vi "MonitorZoomOffset.vi"() -> ()   [LabVIEW 2016]
uses:
  controls/Enum.ctl
  <vilib>/Utility/miscctls.llb/LVPointDoubleTypeDef.ctl
  Course Project/support/Message Queue/Message Cluster.ctl
  <vilib>/Utility/cursorutil.llb/Set Cursor (Icon Pict).vi
  Course Project/support/Message Queue/Message Queue.lvlib
panel:
  out "Line (um)":dbl format="%.2pm"
  in  "Square Zoom":bool
  in  "Apply Old":bool
  in  "Selection Old":T1(radio)
  out "Intensity Graph":dbl[][](graph)
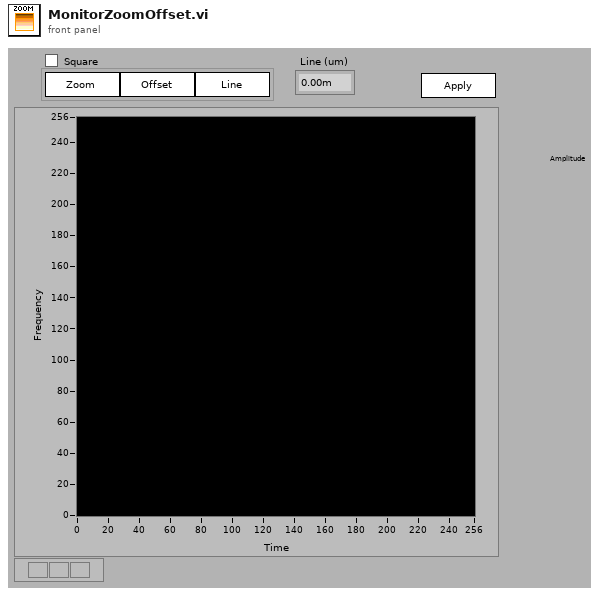
[diagram p1: front panel]
types:
  T1 = enum32{"No Selection", "Zoom", "Offset", "Profile\nProfile"}
  T2 = typedef "Enum.ctl" = enum16{"Init", "Read", "Write"}
  T3 = cluster{"Width":dbl, "Height":dbl, "X Offset":dbl, "Y Offset":dbl, "Angle":dbl, "Pixels/Line":u16, "Lines":u16, "Time/Line":dbl, "Scan Rate":dbl}
  T4 = typedef "LVRectTypeDef.ctl" = cluster{"Left":i16, "Top":i16, "Right":i16, "Bottom":i16}
  T5 = cluster{"Width":i16, "Style":enum32{"Solid", "Dash", "Dot", "DashDot", "DashDotDot"}}
  T6 = cluster{"Width":u16, "Style":enum32{"Solid", "Dash", "Dot", "DashDot", "DashDotDot"}}
  T7 = cluster{"left":i16, "top":i16, "right":i16, "bottom":i16}
  T8 = typedef "Message Queue.lvlib/Message Cluster.ctl" = cluster{"Message":string, "Données de message":variant}
  T9 = typedef "LVPoint32TypeDef.ctl" = cluster{"Horizontal":i32, "Vertical":i32}
  T10 = typedef "LVRangeTypeDef.ctl" = cluster{"Minimum":dbl, "Maximum":dbl, "Increment":dbl, "Minor Increment":dbl, "Start":dbl}
  T11 = typedef "LVBoundsTypeDef.ctl" = cluster{"Width":u32, "Height":u32}
  T12 = typedef "LVPointDoubleTypeDef.ctl" = cluster{"X":dbl, "Y":dbl}
  T13 = cluster{"Left coord px":dbl, "Right coord px":dbl, "Top coord px":dbl, "Bottom coord px":dbl}
  T14 = cluster{"Zoom Center  X um":dbl, "Zoom Center Y um":dbl}
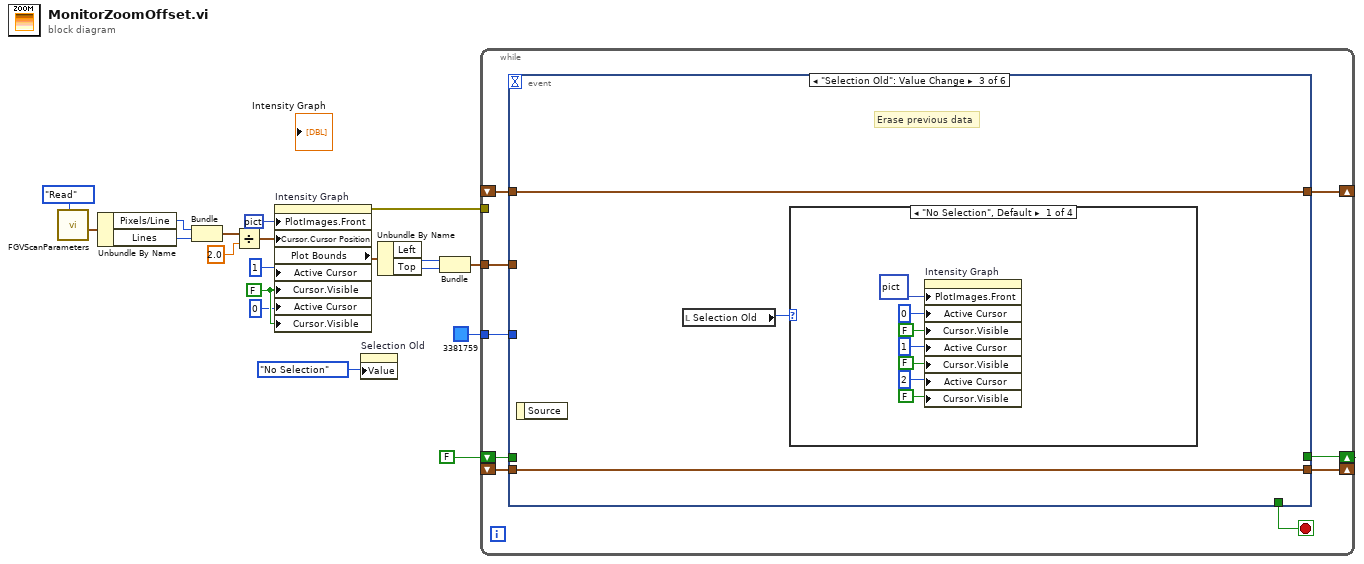
[diagram p0: block diagram]
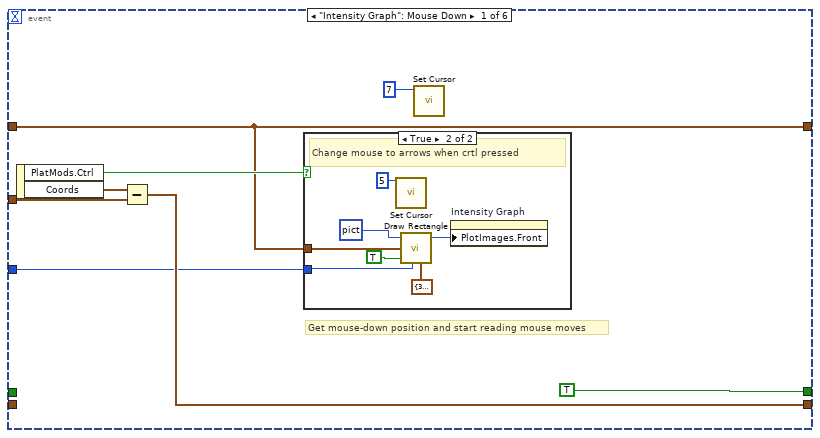
[diagram p2: hidden frame]
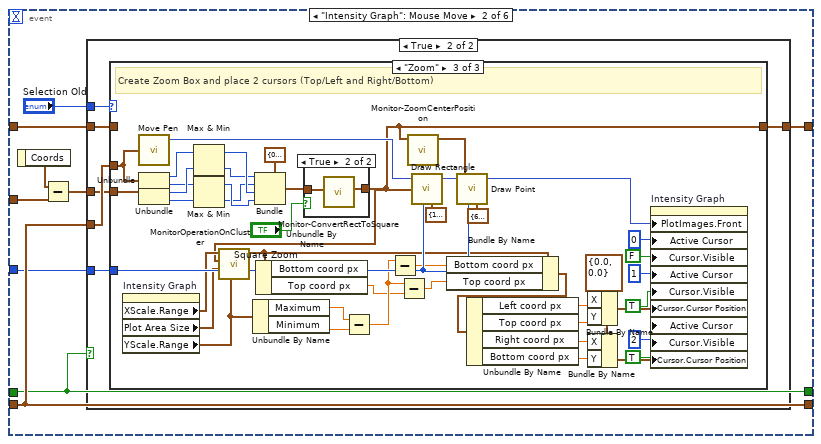
[diagram p4: hidden frame]
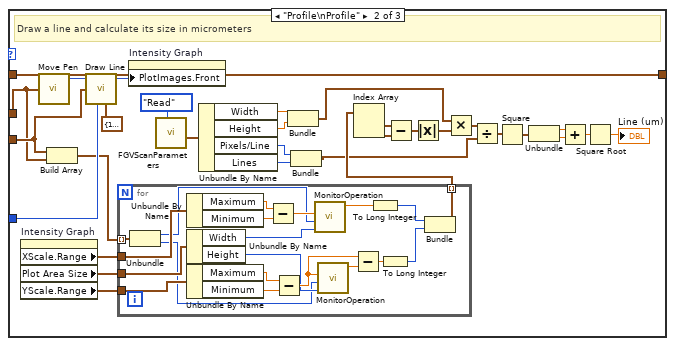
[diagram p7: hidden frame]
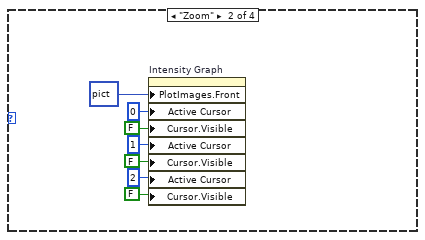
[diagram p9: hidden frame]
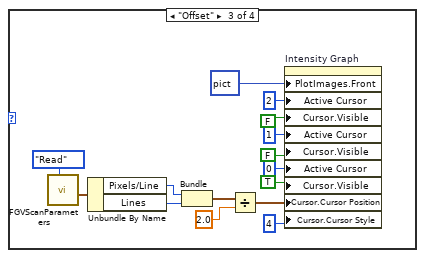
[diagram p10: hidden frame]
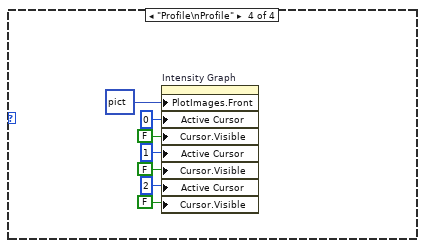
[diagram p11: hidden frame]
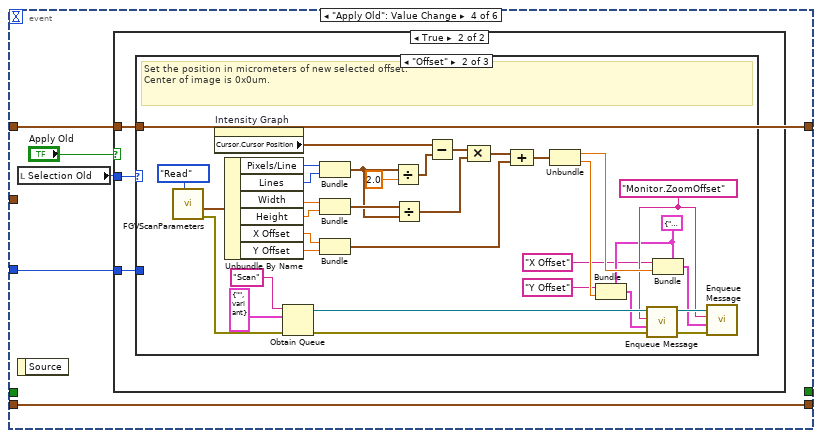
[diagram p12: hidden frame]
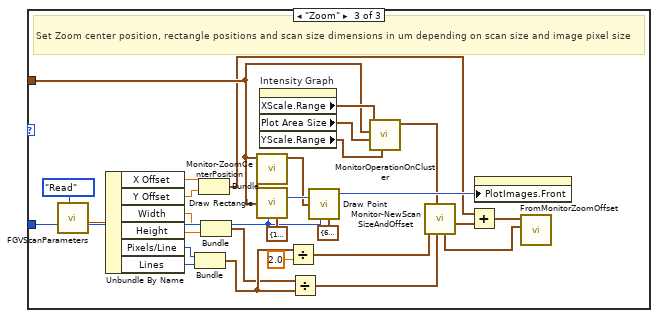
[diagram p15: hidden frame]
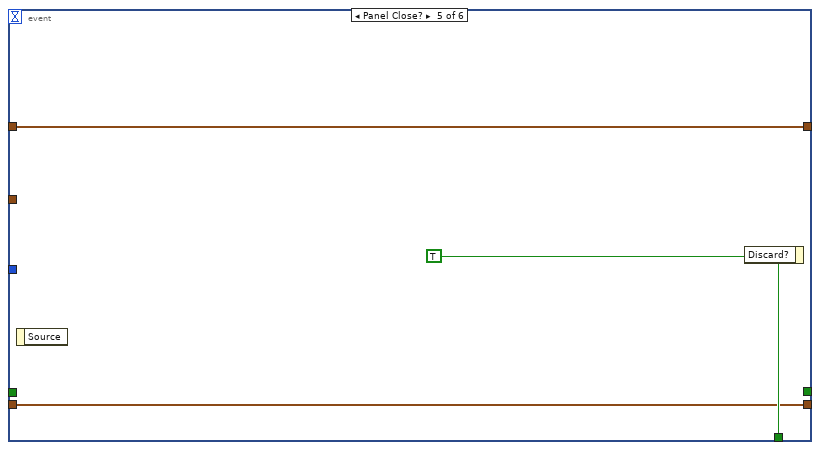
[diagram p16: hidden frame]
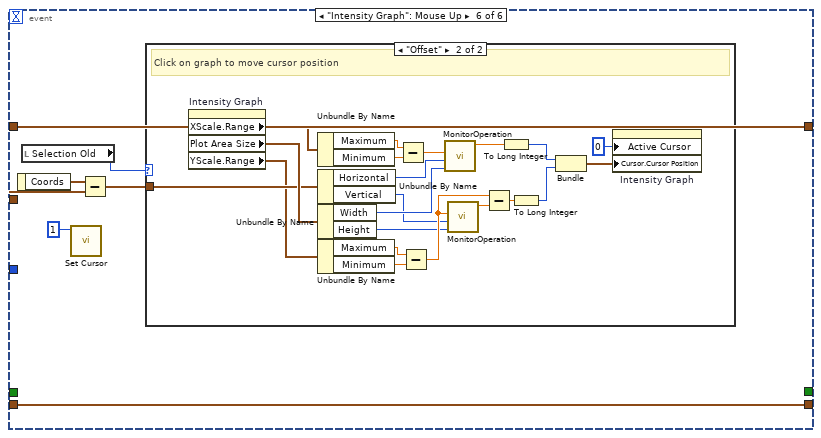
[diagram p17: hidden frame]
diagram:
  w7 = FALSE ("Cursor.Visible")
  n1 = call "FGVScanParameters.vi"("Enum"=Enum."Read") -> ("Scan Parameters Out"=w4:T3)  [unwired: 9 in, 1 out]
  n2 = Unbundle By Name(w4) -> ("Pixels/Line"=w3:u16, "Lines"=w2:u16)
  n3 = Bundle("Pixels/Line"=w3, "Lines"=w2) -> (w1:cluster{"Pixels/Line":u16, "Lines":u16})  [unwired: 1 in]
  n4 = Divide(x=w1, y=2.0) -> (x/y=w8:cluster{"Pixels/Line":dbl, "Lines":dbl})
  n5 = property on="Intensity Graph" class="IntGraph (strict)"("PlotImages.Front"=picture data[5B] ("Plot Images:Front"), "Cursor.Cursor Position"=w8, "Active Cursor"=u32 1, "Cursor.Visible"=w7, "Active Cursor"=u32 0, "Cursor.Visible"=w7) -> (error out=w12:errorcluster, "Plot Bounds"=w11:T4)  [unwired: 2 in, 1 out]
  n6 = property on="Selection Old" class="RadioBtnsControl (strict)"("Value"=T1."No Selection" ("Selection")) -> ()  [unwired: 2 in, 2 out]
  n7 = Unbundle By Name(w11) -> ("Left"=w18:i16, "Top"=w17:i16)
  n8 = Bundle("Left"=w18, "Top"=w17) -> (w15:cluster{"Left":i16, "Top":i16})  [unwired: 1 in]
  n9 = while {
    shift-right: [w28] -> _
    shift-left: _ -> [w27]
    shift-right: [w26] -> _
    shift-left: FALSE -> [w25]
    tunnel: w15 -> [w23]
    tunnel: u32 3381759 ("Line Color 2") -> [w22]
    tunnel: w12 -> [_]
    shift-right: [w21] -> _
    shift-left: _ -> [w20]
    stop <- w24 stop-if-true
    n10 = event shown="[2] \"Selection Old\": Value Change" {
      selector: _ -> [_ _ _ _ _ _]
      dyn-events: _ -> [_ _ _ _ _ _]
      timeout: _ -> [_ _ _ _ _ _]
      tunnel: [w35 w52 w162 w202 w268 w272] -> w28
      tunnel: w27 -> [_ w52 w162 w202 w268 w272]
      tunnel: [TRUE w51 _ _ _ _] -> w26
      tunnel: w25 -> [_ w51 _ _ _ _]
      tunnel: [_ _ _ _ w270 _] -> w24
      tunnel: w23 -> [w34 w48 _ _ _ w274]
      tunnel: w22 -> [w31 w47 _ w203 _ _]
      tunnel: [w29 w45 w161 w200 w269 w271] -> w21
      tunnel: w20 -> [w29 w44 w161 w200 w269 w271]
      event "Intensity Graph": Mouse Down {
        # "Get mouse-down position and start reading mouse moves"
        n11 = event-data() -> ("PlatMods.Ctrl"=w30:bool, "Coords"=w32:T9)  [unwired: 1 in]
        n12 = Subtract(x=w32, y=w34) -> (x-y=w35:T9)
        n13 = case shown="True" w30 {
          tunnel: w31 -> [_ w40]
          tunnel: w29 -> [_ w37]
          frame False {
          }
          frame True {
            # "Change mouse to arrows when crtl pressed"
            n14 = call-poly <vilib>:"Set Cursor.vi"("icon"=u16 5) -> ()  [unwired: 9 in, 2 out]
            n15 = call <vilib>:"Draw Rectangle.vi"("picture"=picture data[5B], "rect"=w37, "fill?(F)"=TRUE, "color(black)"=w40, "pen"=T5 {"Width"=3, "Style"=enum."Solid"}) -> ("new picture"=w38:picture)  [unwired: 4 in]
            n16 = property on="Intensity Graph" class="IntGraph (strict)"("PlotImages.Front"=w38) -> ()  [unwired: 2 in, 2 out]
          }
        }
        n17 = call-poly <vilib>:"Set Cursor.vi"("icon"=u16 7) -> ()  [unwired: 9 in, 2 out]
      }
      event "Intensity Graph": Mouse Move {
        n18 = event-data() -> ("Coords"=w50:T9)  [unwired: 1 in]
        n19 = Subtract(x=w50, y=w48) -> (x-y=w49:T9)
        n20 = case shown="True" w51 {
          tunnel: w52 -> [_ w59]
          tunnel: w49 -> [_ w58]
          tunnel: "Selection Old" -> [_ w57]
          tunnel: w47 -> [_ w56]
          tunnel: [w53 w55] -> w45
          tunnel: w44 -> [w53 w54]
          frame False {
          }
          frame True {
            n21 = case shown="\"Zoom\"" w57 {
              tunnel: w59 -> [_ w75 w156]
              tunnel: w58 -> [_ w76 w154]
              tunnel: w56 -> [_ w88 w155]
              tunnel: [w60 w87 w114] -> w55
              tunnel: w54 -> [w60 w87 _]
              frame "No Selection", Default {
              }
              frame "Profile\nProfile" {
                # "Draw a line and calculate its size in micrometers"
                n22 = property on="Intensity Graph" class="IntGraph (strict)"() -> ("XScale.Range"=w73:T10, "Plot Area Size"=w72:T11, "YScale.Range"=w69:T10)  [unwired: 2 in, 2 out]
                n23 = call <vilib>:"Move Pen.vi"("new position"=w75) -> ("new picture"=w91:picture)  [unwired: 4 in]
                n24 = Build Array(w76, w75) -> (w74:T9[])
                n25 = call <vilib>:"Draw Line.vi"("picture"=w91, "end point"=w76, "color(black)"=w88, "pen"=T6 {"Width"=1, "Style"=enum."Solid"}) -> ("new picture"=w89:picture)  [unwired: 5 in]
                n26 = for {
                  tunnel: w74 -> [w95] mode=indexing
                  tunnel: w73 -> [w96]
                  tunnel: w69 -> [w97]
                  tunnel: w72 -> [w98]
                  tunnel: [w92] -> w70 mode=indexing
                  n27 = Unbundle(w95) -> ("Horizontal"=w94:i32, "Vertical"=w93:i32)
                  n28 = Unbundle By Name(w96) -> ("Maximum"=w108:dbl, "Minimum"=w109:dbl)
                  n29 = Unbundle By Name(w98) -> ("Width"=w104:u32, "Height"=w100:u32)
                  n30 = Unbundle By Name(w97) -> ("Maximum"=w110:dbl, "Minimum"=w111:dbl)
                  n31 = Subtract(x=w108, y=w109) -> (x-y=w102:dbl)
                  n32 = Subtract(x=w110, y=w111) -> (x-y=w101:dbl)
                  n33 = call "MonitorOperation.vi"("Width"=w104, "Right"=w94, "Max - Min"=w102) -> ("Conversion"=w103:dbl)  [unwired: 8 in]
                  n34 = call "MonitorOperation.vi"("Width"=w100, "Right"=w93, "Max - Min"=w101) -> ("Conversion"=w99:dbl)  [unwired: 8 in]
                  n35 = Subtract(x=w101, y=w99) -> (x-y=w106:dbl)
                  n36 = To Long Integer(number=w103) -> (32bit integer=w107:i32)
                  n37 = To Long Integer(number=w106) -> (32bit integer=w105:i32)
                  n38 = Bundle(w107, w105) -> (w92:cluster{i32, i32})  [unwired: 1 in]
                }
                n39 = property on="Intensity Graph" class="IntGraph (strict)"("PlotImages.Front"=w89) -> ()  [unwired: 2 in, 2 out]
                n40 = call "FGVScanParameters.vi"("Enum"=Enum."Read") -> ("Scan Parameters Out"=w67:T3)  [unwired: 9 in, 1 out]
                n41 = Unbundle By Name(w67) -> ("Width"=w66:dbl, "Height"=w65:dbl, "Pixels/Line"=w64:u16, "Lines"=w63:u16)
                n42 = Bundle("Width"=w66, "Height"=w65) -> (w62:cluster{"Width":dbl, "Height":dbl})  [unwired: 1 in]
                n43 = Bundle("Pixels/Line"=w64, "Lines"=w63) -> (w61:cluster{"Pixels/Line":u16, "Lines":u16})  [unwired: 1 in]
                n44 = Index Array(array=w70) -> (element #1=w78:cluster{i32, i32}, element #2=w77:cluster{i32, i32})  [unwired: 2 in]
                n45 = Subtract(x=w78, y=w77) -> (x-y=w79:cluster{i32, i32})
                n46 = Absolute Value(x=w79) -> (abs(x)=w71:cluster{i32, i32})
                n47 = Multiply(x=w62, y=w71) -> (x*y=w85:cluster{dbl, dbl})
                n48 = Divide(x=w85, y=w61) -> (x/y=w84:cluster{dbl, dbl})
                n49 = Square(x=w84) -> (x^2=w83:cluster{dbl, dbl})
                n50 = Unbundle(w83) -> (w82:dbl, w81:dbl)
                n51 = Add(x=w82, y=w81) -> (x+y=w86:dbl)
                n52 = Square Root(x=w86) -> (sqrt(x)=→"Line (um)":dbl)
              }
              frame "Zoom" {
                w129 = T12 {"X"=0.0, "Y"=0.0} ("Cursor.Cursor Position")
                # "Create Zoom Box and place 2 cursors (Top/Left and Right/Bottom)"
                n53 = property on="Intensity Graph" class="IntGraph (strict)"() -> ("XScale.Range"=w116:T10, "Plot Area Size"=w115:T11, "YScale.Range"=w113:T10)  [unwired: 2 in, 2 out]
                n54 = call <vilib>:"Move Pen.vi"("new position"=w156) -> ("new picture"=w153:picture)  [unwired: 4 in]
                n55 = Unbundle(w156) -> ("Horizontal"=w150:i32, "Vertical"=w147:i32)
                n56 = Unbundle(w154) -> ("Horizontal"=w149:i32, "Vertical"=w146:i32)
                n57 = Max & Min(x=w150, y=w149) -> (max(x,y)=w148:i32, min(x,y)=w144:i32)
                n58 = Max & Min(x=w147, y=w146) -> (max(x,y)=w145:i32, min(x,y)=w143:i32)
                n59 = Unbundle By Name(w113) -> ("Maximum"=w118:dbl, "Minimum"=w117:dbl)
                n60 = Bundle(cluster=T7 {"left"=0, "top"=0, "right"=0, "bottom"=0} ("rect"), "left"=w144, "top"=w143, "right"=w148, "bottom"=w145) -> (w142:T7)
                n61 = case shown="True" "Square Zoom" {
                  tunnel: w142 -> [w158 w160]
                  tunnel: [w158 w159] -> w114
                  frame False {
                  }
                  frame True {
                    n62 = call "Monitor-ConvertRectToSquare.vi"("Rect coords in"=w160) -> ("Square coords out"=w159:T7)  [unwired: 10 in]
                  }
                }
                n63 = call "MonitorOperationOnCluster.vi"("YScale.Range"=w113, "Plot Area Size"=w115, "Original Zoom rect coords"=w114, "XScale.Range"=w116) -> ("Rect coords  graph scale"=w124:T13)  [unwired: 7 in]
                n64 = Unbundle By Name(w124) -> ("Bottom coord px"=w123:dbl, "Top coord px"=w121:dbl)
                n65 = Subtract(x=w118, y=w117) -> (x-y=w122:dbl)
                n66 = Subtract(x=w122, y=w123) -> (x-y=w119:dbl)
                n67 = Subtract(x=w122, y=w121) -> (x-y=w120:dbl)
                n68 = call "Monitor-ZoomCenterPosition.vi"("Zoom rect coords"=w114) -> ("Zoom Center Coord"=w140:cluster{" X":dbl, "Y":dbl})  [unwired: 10 in]
                n69 = call <vilib>:"Draw Rectangle.vi"("picture"=w153, "rect"=w114, "color(black)"=w155, "pen"=T6 {"Width"=1, "Style"=enum."Dot"}) -> ("new picture"=w139:picture)  [unwired: 5 in]
                n70 = Bundle By Name(cluster=w124, "Bottom coord px"=w119, "Top coord px"=w120) -> (w112:T13)
                n71 = call <vilib>:"Draw Point.vi"("picture"=w139, "point(x,y)"=w140, "color(black)"=w155, "pen"=T6 {"Width"=6, "Style"=enum."Solid"}) -> ("new picture"=w132:picture)  [unwired: 5 in]
                n72 = Unbundle By Name(w112) -> ("Left coord px"=w137:dbl, "Top coord px"=w130:dbl, "Right coord px"=w128:dbl, "Bottom coord px"=w127:dbl)
                n73 = Bundle By Name(cluster=w129, "X"=w137, "Y"=w130) -> (w131:T12)
                n74 = Bundle By Name(cluster=w129, "X"=w128, "Y"=w127) -> (w157:T12)
                n75 = property on="Intensity Graph" class="IntGraph (strict)"("PlotImages.Front"=w132, "Active Cursor"=u32 0, "Cursor.Visible"=FALSE, "Active Cursor"=u32 1, "Cursor.Visible"=TRUE, "Cursor.Cursor Position"=w131, "Active Cursor"=u32 2, "Cursor.Visible"=TRUE, "Cursor.Cursor Position"=w157) -> ()  [unwired: 2 in, 2 out]
              }
            }
          }
        }
      }
      event "Selection Old": Value Change {
        # "Erase previous data"
        # "Radio Box functions"
        n76 = event-data() -> ()  [unwired: 1 in, 1 out]
        n77 = local read "Selection Old"() -> (w163:T1)
        n78 = case shown="\"No Selection\", Default" w163 {
          frame "No Selection", Default {
            # "Erase previous data for no selection"
            n79 = property on="Intensity Graph" class="IntGraph (strict)"("PlotImages.Front"=picture data[5B] ("Plot Images:Front"), "Active Cursor"=0 ("Cursor.Cursor Index"), "Cursor.Visible"=FALSE, "Active Cursor"=u32 1, "Cursor.Visible"=FALSE, "Active Cursor"=u32 2, "Cursor.Visible"=FALSE) -> ()  [unwired: 2 in, 2 out]
          }
          frame "Zoom" {
            # "Erase previous data for Zoom"
            n80 = property on="Intensity Graph" class="IntGraph (strict)"("PlotImages.Front"=picture data[5B] ("Plot Images:Front"), "Active Cursor"=0 ("Cursor.Cursor Index"), "Cursor.Visible"=FALSE, "Active Cursor"=u32 1, "Cursor.Visible"=FALSE, "Active Cursor"=u32 2, "Cursor.Visible"=FALSE) -> ()  [unwired: 2 in, 2 out]
          }
          frame "Offset" {
            # "Display the offset cursor in the center of graph and erase previous data"
            n81 = call "FGVScanParameters.vi"("Enum"=Enum."Read") -> ("Scan Parameters Out"=w181:T3)  [unwired: 9 in, 1 out]
            n82 = Unbundle By Name(w181) -> ("Pixels/Line"=w180:u16, "Lines"=w179:u16)
            n83 = Bundle("Pixels/Line"=w180, "Lines"=w179) -> (w178:cluster{"Pixels/Line":u16, "Lines":u16})  [unwired: 1 in]
            n84 = Divide(x=w178, y=2.0) -> (x/y=w184:cluster{"Pixels/Line":dbl, "Lines":dbl})
            n85 = property on="Intensity Graph" class="IntGraph (strict)"("PlotImages.Front"=picture data[5B] ("Plot Images:Front"), "Active Cursor"=2 ("Cursor.Cursor Index"), "Cursor.Visible"=FALSE, "Active Cursor"=u32 1, "Cursor.Visible"=FALSE, "Active Cursor"=u32 0, "Cursor.Visible"=TRUE, "Cursor.Cursor Position"=w184, "Cursor.Cursor Style"=u8 4) -> ()  [unwired: 2 in, 2 out]
          }
          frame "Profile\nProfile" {
            # "Erase previous data for distance measurement"
            n86 = property on="Intensity Graph" class="IntGraph (strict)"("PlotImages.Front"=picture data[5B] ("Plot Images:Front"), "Active Cursor"=0 ("Cursor.Cursor Index"), "Cursor.Visible"=FALSE, "Active Cursor"=u32 1, "Cursor.Visible"=FALSE, "Active Cursor"=u32 2, "Cursor.Visible"=FALSE) -> ()  [unwired: 2 in, 2 out]
          }
        }
      }
      event "Apply Old": Value Change {
        n87 = local read "Selection Old"() -> (w201:T1)
        n88 = event-data() -> ()  [unwired: 1 in, 1 out]
        n89 = case shown="True" "Apply Old" {
          tunnel: w203 -> [_ w207]
          tunnel: w201 -> [_ w206]
          tunnel: w200 -> [_ w205]
          frame False {
          }
          frame True {
            n90 = case shown="\"Offset\"" w206 {
              tunnel: w207 -> [_ _ w263]
              tunnel: w205 -> [_ _ w256]
              frame "No Selection", Default {
              }
              frame "Offset" {
                w211 = cluster{"ControlName":string, "Value":dbl} {"ControlName"="", "Value"=0.0} ("Data")
                w212 = "Monitor.ZoomOffset" ("Message")
                # "Set the position in micrometers of new selected offset. \nCenter of image is 0x0um."
                n91 = call "FGVScanParameters.vi"("Enum"=Enum."Read") -> ("error out"=w216:errorcluster, "Scan Parameters Out"=w231:T3)  [unwired: 9 in]
                n92 = property on="Intensity Graph" class="IntGraph (strict)"() -> ("Cursor.Cursor Position"=w234:T12)  [unwired: 2 in, 2 out]
                n93 = Unbundle By Name(w231) -> ("Pixels/Line"=w227:u16, "Lines"=w226:u16, "Width"=w230:dbl, "Height"=w229:dbl, "X Offset"=w222:dbl, "Y Offset"=w221:dbl)
                n94 = Obtain Queue(name (unnamed)="Scan" ("QueueName"), element data type=T8 {"Message"="", "Données de message"=variant} ("Cluster Message"), error in (no error)=w216) -> (queue out=w238:refnum<queue>, error out=w217:errorcluster)  [unwired: 2 in, 1 out]
                n95 = Bundle("Pixels/Line"=w227, "Lines"=w226) -> (w223:cluster{"Pixels/Line":u16, "Lines":u16})  [unwired: 1 in]
                n96 = Bundle("Width"=w230, "Height"=w229) -> (w228:cluster{"Width":dbl, "Height":dbl})  [unwired: 1 in]
                n97 = Bundle("X Offset"=w222, "Y Offset"=w221) -> (w220:cluster{"X Offset":dbl, "Y Offset":dbl})  [unwired: 1 in]
                n98 = Divide(x=w223, y=2.0) -> (x/y=w235:cluster{"Pixels/Line":dbl, "Lines":dbl})
                n99 = Divide(x=w228, y=w223) -> (x/y=w224:cluster{dbl, dbl})
                n100 = Subtract(x=w234, y=w235) -> (x-y=w225:T12)
                n101 = Compound Arithmetic op=MULTIPLY(w225, w224) -> (w233:T12)
                n102 = Compound Arithmetic op=ADD(w233, w220) -> (w214:T12)
                n103 = Unbundle(w214) -> ("Cursor X"=w237:dbl, "Cursor Y"=w210:dbl)
                n104 = Bundle(cluster=w211, "ControlName"="Y Offset" ("Message"), "Value"=w210) -> (w213:cluster{"ControlName":string, "Value":dbl})
                n105 = call "Enqueue Message.vi"("Data"=w213, "Message"=w212, "Queue"=w238) -> ("Queue dup."=w239:refnum<queue>)  [unwired: 7 in, 1 out]
                n106 = Bundle(cluster=w211, "ControlName"="X Offset" ("Message"), "Value"=w237) -> (w215:cluster{"ControlName":string, "Value":dbl})
                n107 = call "Enqueue Message.vi"("error in"=w217, "Data"=w215, "Message"=w212, "Queue"=w239) -> ()  [unwired: 6 in, 2 out]
              }
              frame "Zoom" {
                # "Set Zoom center position, rectangle positions and scan size dimensions in um depending on scan size and image pixel size"
                n108 = call "FGVScanParameters.vi"("Enum"=Enum."Read") -> ("Scan Parameters Out"=w252:T3)  [unwired: 9 in, 1 out]
                n109 = Unbundle By Name(w252) -> ("X Offset"=w244:dbl, "Y Offset"=w243:dbl, "Width"=w247:dbl, "Height"=w246:dbl, "Pixels/Line"=w249:u16, "Lines"=w250:u16)
                n110 = Bundle("Pixels/Line"=w249, "Lines"=w250) -> (w248:cluster{"Pixels/Line":u16, "Lines":u16})  [unwired: 1 in]
                n111 = Bundle("X Offset"=w244, "Y Offset"=w243) -> (w242:cluster{"X Offset":dbl, "Y Offset":dbl})  [unwired: 1 in]
                n112 = Bundle("Width"=w247, "Height"=w246) -> (w245:cluster{"Width":dbl, "Height":dbl})  [unwired: 1 in]
                n113 = call "Monitor-ZoomCenterPosition.vi"("Zoom rect coords"=w256) -> ("Zoom Center Coord"=w264:cluster{" X":dbl, "Y":dbl})  [unwired: 10 in]
                n114 = call <vilib>:"Draw Rectangle.vi"("rect"=w256, "color(black)"=w263, "pen"=T5 {"Width"=1, "Style"=enum."Dot"}) -> ("new picture"=w266:picture)  [unwired: 6 in]
                n115 = property on="Intensity Graph" class="IntGraph (strict)"() -> ("XScale.Range"=w257:T10, "Plot Area Size"=w255:T11, "YScale.Range"=w254:T10)  [unwired: 2 in, 2 out]
                n116 = Divide(x=w248, y=2.0) -> (x/y=w260:cluster{"Pixels/Line":dbl, "Lines":dbl})
                n117 = Divide(x=w245, y=w248) -> (x/y=w258:cluster{dbl, dbl})
                n118 = call <vilib>:"Draw Point.vi"("picture"=w266, "point(x,y)"=w264, "color(black)"=w263, "pen"=T6 {"Width"=6, "Style"=enum."Solid"}) -> ("new picture"=w262:picture)  [unwired: 5 in]
                n119 = call "MonitorOperationOnCluster.vi"("YScale.Range"=w254, "Plot Area Size"=w255, "Original Zoom rect coords"=w256, "XScale.Range"=w257) -> ("Rect coords  graph scale"=w253:T13)  [unwired: 7 in]
                n120 = call "Monitor-NewScanSizeAndOffset.vi"("um/px"=w258, "Zoom Rect coords px"=w253, "Scan Size Center pixels"=w260) -> ("Zoom Center coords um"=w261:T14, "New Scan Size"=w240:cluster{"Width um":dbl, " Height um":dbl})  [unwired: 7 in]
                n121 = Add(x=w242, y=w261) -> (x+y=w241:cluster{dbl, dbl})
                n122 = property on="Intensity Graph" class="IntGraph (strict)"("PlotImages.Front"=w262) -> ()  [unwired: 2 in, 2 out]
                n123 = call "FromMonitorZoomOffset.vi"("Size"=w240, "Offset"=w241) -> ()  [unwired: 10 in]
              }
            }
          }
        }
      }
      event Panel Close? {
        w270 = TRUE ("stop")
        n124 = event-data() -> ()  [unwired: 1 in, 1 out]
        n125 = event-data("Discard?"=w270) -> ()  [unwired: 1 in, 1 out]
      }
      event "Intensity Graph": Mouse Up {
        n126 = event-data() -> ("Coords"=w276:T9)  [unwired: 1 in]
        n127 = local read "Selection Old"() -> (w277:T1)
        n128 = call-poly <vilib>:"Set Cursor.vi"("icon"=u16 1) -> ()  [unwired: 9 in, 2 out]
        n129 = Subtract(x=w276, y=w274) -> (x-y=w275:T9)
        n130 = case shown="\"Offset\"" w277 {
          tunnel: w275 -> [_ w280]
          frame "No Selection", Default {
          }
          frame "Offset" {
            # "Click on graph to move cursor position"
            n131 = property on="Intensity Graph" class="IntGraph (strict)"() -> ("XScale.Range"=w282:T10, "Plot Area Size"=w281:T11, "YScale.Range"=w278:T10)  [unwired: 2 in, 2 out]
            n132 = Unbundle By Name(w282) -> ("Maximum"=w294:dbl, "Minimum"=w295:dbl)
            n133 = Unbundle By Name(w280) -> ("Horizontal"=w290:i32, "Vertical"=w285:i32)
            n134 = Unbundle By Name(w281) -> ("Width"=w289:u32, "Height"=w284:u32)
            n135 = Unbundle By Name(w278) -> ("Maximum"=w296:dbl, "Minimum"=w297:dbl)
            n136 = Subtract(x=w294, y=w295) -> (x-y=w287:dbl)
            n137 = Subtract(x=w296, y=w297) -> (x-y=w286:dbl)
            n138 = call "MonitorOperation.vi"("Width"=w289, "Right"=w290, "Max - Min"=w287) -> ("Conversion"=w288:dbl)  [unwired: 8 in]
            n139 = call "MonitorOperation.vi"("Width"=w284, "Right"=w285, "Max - Min"=w286) -> ("Conversion"=w283:dbl)  [unwired: 8 in]
            n140 = Subtract(x=w286, y=w283) -> (x-y=w292:dbl)
            n141 = To Long Integer(number=w288) -> (32bit integer=w293:i32)
            n142 = To Long Integer(number=w292) -> (32bit integer=w291:i32)
            n143 = Bundle(w293, w291) -> (w279:cluster{i32, i32})  [unwired: 1 in]
            n144 = property on="Intensity Graph" class="IntGraph (strict)"("Active Cursor"=u32 0, "Cursor.Cursor Position"=w279) -> ()  [unwired: 2 in, 2 out]
          }
        }
      }
    }
  }
